vi "Normalize Path String.vi"(10 "Import String":string) -> (2 "Normalized Path":string)   [LabVIEW 2020, in "LV-Protoc.lvlib" / "ProtoParser.lvclass"]
uses:
  ProtoParser.lvclass
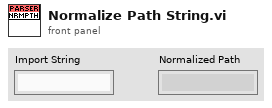
[diagram p1: front panel]
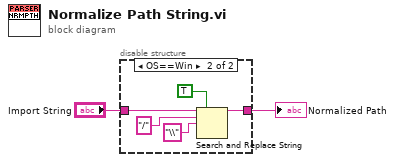
[diagram p0: block diagram]
diagram:
  n1 = disable-structure shown="OS==Win" {
    disable-tunnel: "Import String" -> [w3 w8]
    disable-tunnel: [w3 w4] -> w1
    frame condition #0 {
    }
    frame condition #1 (active) {
      n2 = Search and Replace String(replace all?=TRUE ("replace all? (F)"), input string=w8, search string="/", replace string="\\" ("search string")) -> (result string=w4:string)  [unwired: 4 in, 3 out]
    }
  }
  "Normalized Path" <- w1
